vi "GateControlLoop.vi"   [LabVIEW 2014, in "GateLib.lvlib"]
uses:
  GateLib.lvlib
  GateRefs.ctl
  <vilib>/Rock Robotics/WPI/Solenoid/WPI_SolenoidValue.ctl
  <vilib>/Rock Robotics/WPI/Solenoid/WPI_SolenoidSetEnum.vi
types:
  T1 = typedef "GateLib.lvlib/GateRefs.ctl" = enum16{"GateCyl"}
  T2 = typedef "WPI_SolenoidDevRef.ctl" = cluster{"DevStatus":errorcluster, "Pneumatics Control Module":u8, "Forward Solenoid Channel":T3, "Reverse Solenoid Channel":T3}
  T3 = typedef "WPI_SolenoidChannel.ctl" = enum8{"Solenoid 0", "Solenoid 1", "Solenoid 2", "Solenoid 3", "Solenoid 4", "Solenoid 5", "Solenoid 6", "Solenoid 7", "Invalid"}
  T4 = typedef "WPI_SolenoidValue.ctl" = enum16{"Off", "On", "Forward", "Reverse"}
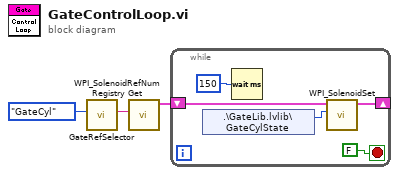
[diagram p0: block diagram]
diagram:
  n1 = call "GateRefSelector.vi"("GateRefs"=GateRefs."GateCyl") -> ("Refnum"=w3:string)  [unwired: 10 in]
  n2 = call <vilib>:"WPI_SolenoidRefNum Registry Get.vi"("refnum name"=w3) -> ("SolenoidDevRef"=w1:T2)  [unwired: 9 in, 1 out]
  n3 = while {
    shift-right: [w6] -> _
    shift-left: w1 -> [w7]
    stop <- FALSE stop-if-true
    n4 = shared-variable ".\\GateLib.lvlib\\GateCylState"() -> (w8:T4)  [unwired: 1 in, 1 out]
    n5 = Wait (ms)(milliseconds to wait=u32 150) -> ()  [unwired: 1 out]
    n6 = call-poly <vilib>:"WPI_SolenoidSet.vi"("Value"=w8, "SolenoidDevRef"=w7) -> ("SolenoidDevRef"=w6:T2)  [unwired: 8 in, 1 out]
  }
